vi "RT Main.vi"() -> ()   [LabVIEW 2014]
uses:
  <vilib>/NI/cRIO Wfm/cRIO Wfm.lvlib
  <vilib>/NI/cRIO Wfm/AcqRead(Wfm).vi
  <vilib>/rvi/interface/nirviOpenFPGA/nirviOpenFPGA.xnode
  <vilib>/rvi/interface/nirviMethod/nirviMethod.xnode
  <vilib>/FPGAPlugInAG/Dynamic/niLvFpga_Reset_Dynamic.vi
  <vilib>/FPGAPlugInAG/Dynamic/niLvFpga_Run_Dynamic.vi
  <vilib>/rvi/interface/nirviCloseFPGA/nirviCloseFPGA.xnode
  <vilib>/addons/Sound and Vibration/svt_Calibration/SoundVib_Calibration.lvlib
  <vilib>/addons/Sound and Vibration/svt_Calibration/SVL Scale Voltage to EU (N Ch - 1 Info).vi
  <vilib>/addons/_NISVFA/_Baseband FFT/SVFA Power Spectrum (N Ch).vi
  <vilib>/addons/_NISVFA/_Zoom FFT/SVFA Zoom Power Spectrum (N Ch).vi
  <vilib>/addons/_NISVFA/_Subset FFT/SVFA Power Spectrum Subset (N Ch).vi
  <vilib>/addons/_NISVFA/_Baseband FFT/SVFA FFT Spectrum (Mag-Phase) (N Ch).vi
  <vilib>/addons/_NISVFA/_Zoom FFT/SVFA Zoom FFT Spectrum (Mag-Phase) (N Ch).vi
  <vilib>/addons/_NISVFA/_Subset FFT/SVFA FFT Spectrum Subset (Mag-Phase) (N Ch).vi
  <vilib>/addons/_NISVFA/_Baseband FFT/SVFA Power Spectral Density (N Ch).vi
  <vilib>/addons/_NISVFA/_Zoom FFT/SVFA Zoom Power Spectral Density (N Ch).vi
  <vilib>/addons/_NISVFA/_Subset FFT/SVFA Power Spectral Density Subset (N Ch).vi
  <vilib>/NI/cRIO Wfm/ChannelConfig.ctl
  <vilib>/NI/cRIO Wfm/DynamicFPGAref.ctl
  <vilib>/FPGAPlugInAG/Dynamic/niLvFpga_Close_Dynamic.vi
  FPGA Bitfiles/SOMHands-OnExerc_FPGATarget_FPGAMainSPIAPI_7cwEv4E7lq8.lvbitx
  <vilib>/FPGAPlugInAG/sbRIO-9651/niLvFpga_Open_sbRIO-9651.vi
  <vilib>/rvi/interface/common/dynamic/niFpgaDynamicAddResources.vi
  <vilib>/addons/_NISVFA/_Shared subVIs/Controls/svc_Window.ctl
  <vilib>/addons/_NISVFA/_Shared subVIs/Controls/svc_Engineering Units Text Ring.ctl
  <vilib>/addons/_NISVFA/_Shared subVIs/Controls/svc_Weighting Filter Text Ring.ctl
  <vilib>/addons/_NISVFA/_Shared subVIs/Controls/svc_Channel Info.ctl
panel:
  in  "channel info":T1={"sensor sensitivity [mV/EU]"=1000.0, "engineering units"=1, "dB reference [EU]"=1.0, "custom label"="EU", "weighting filter"=0, "pregain [dB]"=0.0} {"pregain [dB]" format="%.2f"; "weighting filter" items=["Linear", "A-weighting", "B-weighting", "C-weighting", "ITU-R 468-4", "Dolby", "CCITT", "C-message", "Wb", "Wc", "Wd", "We", "Wf", "Wh", "Wj", "Wk", "Wm", "AES17 20 kHz lowpass", "AES17 40 kHz lowpass", "AES17 20 kHz highpass", "AES17 40 kHz highpass"]; "dB reference [EU]" format="%^.1e"; "engineering units" items=["custom..."=0, "V"=1, "A"=21, "Pa"=2, "N"=20, "g"=3, "m/s^2"=4, "m/s"=5, "m"=6, "mm/s"=12, "mm"=13, "micron/s"=14, "micron"=15, "in/s^2"=7, "in/s"=8, "in"=9, "mil/s"=10, "mil"=11, "rad/s^2"=16, "rad/s"=17, "rad"=18, "deg/s^2"=26, "deg/s"=27, "deg"=28, "RPM"=22, "cycle/s^2"=23, "Hz"=24, "cycle"=25, "strain"=19]; "sensor sensitivity [mV/EU]" format="%.2f"}
  in  "scan rate [S/s]":u32=25000
  in  "quit":bool
  in  "window":T4=1 items=["None"=0, "Hanning"=1, "Hamming"=2, "Blackman-Harris"=3, "Exact Blackman"=4, "Blackman"=5, "Flat Top"=6, "4 Term B-Harris "=7, "7 Term B-Harris"=8, "Low Sidelobe"=9, "Force"=64, "Exponential"=65, "Blackman Nuttall"=11, "Triangle"=30, "Bartlett-Hanning"=31, "Bohman"=32, "Parzen"=33, "Welch"=34, "Kaiser"=60, "Dolph-Chebyshev"=61, "Gaussian"=62]
  in  "Graph Tab Control":T5(tab)
  out "Power spectrum":cluster{"f0":dbl, "df":dbl, "magnitude":dbl[]}[](graph)
  out "Phase":cluster{"f0":dbl, "df":dbl, "phase":dbl[]}[](graph)
  out "Magnitude":cluster{"f0":dbl, "df":dbl, "magnitude":dbl[]}[](graph)
  out "PSD":cluster{"f0":dbl, "df":dbl, "magnitude":dbl[]}[](graph)
  in  "dB On":bool=TRUE
  in  "FFT Type":enum32{"Baseband", "Zoom", "Subset"}(tab)
  out "frequency resolution [Hz]":dbl=50.0 format="%.2f"
  out "time record [ms]":dbl=20.0 format="%.2f"
  in  "zoom settings":T6={"frequency range"={"start frequency"=500.0, "stop frequency"=2000.0}, "window"=enum."Hanning", "number of lines"=400, "% overlap"=0.0} {"% overlap" min=0.0 max=99.0 step=10.0 format="%.2f"; "number of lines" min=1 step=1; "frequency range"."stop frequency" min=0.0 format="%.2f"; "frequency range"."start frequency" min=0.0 format="%.2f"}
  out "zoom FFT":dbl=2.500000055879356 format="%.2f"
  out "baseband FFT":dbl=50.0 format="%.2f"
  out "frequency resolution [Hz] Subset":dbl format="%.2f"
  out "time record [ms] Subset":dbl format="%.2f"
  in  "frequency range 2":T7={"start frequency"=200.0, "stop frequency"=2000.0} {"stop frequency" min=0.0 format="%.2f"; "start frequency" min=0.0 format="%.2f"}
  in  "number of samples":i32=2000 min=128
  out "averages completed":dbl
  out "done":bool
  in  "averaging mode":T8(ring)=enum."RMS averaging"
  in  "number of averages":u32=10
  in  "linear mode":enum16{"One shot", "Auto restart"}(ring)=enum."Auto restart"
  in  "weighting mode":enum16{"Linear", "Exponential"}(ring)=enum."Exponential"
  in  "restart 2":bool
  in  "Samples per Channel":i32=1000
  # "Channel Settings"
  # "Averaging Settings"
  # "Analysis Settings"
  # "VI Controls"
  # "Increase number of samples to improve frequency resolution (for a given sampling frequency)"
  # "frequency resolution [Hz]"
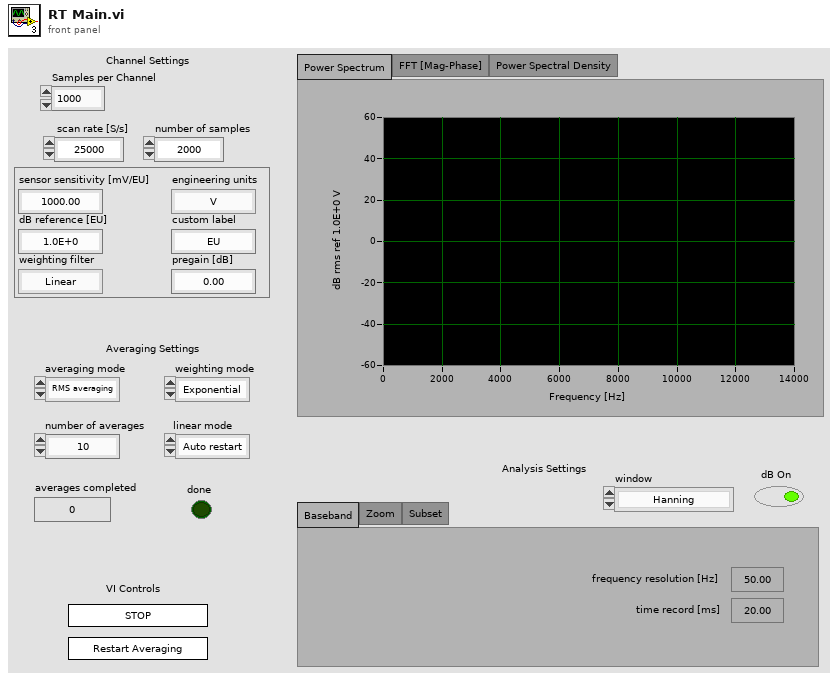
[diagram p1: front panel]
types:
  T1 = typedef "svc_Channel Info.ctl" = cluster{"sensor sensitivity [mV/EU]":dbl, "engineering units":T2, "dB reference [EU]":dbl, "custom label":string, "weighting filter":T3, "pregain [dB]":dbl}
  T2 = typedef "svc_Engineering Units Text Ring.ctl" = u16
  T3 = typedef "svc_Weighting Filter Text Ring.ctl" = u16
  T4 = typedef "svc_Window.ctl" = u32
  T5 = enum32{"Power Spectrum", "FFT [Mag-Phase]", "Power Spectral Density"}
  T6 = cluster{"frequency range":cluster{"start frequency":dbl, "stop frequency":dbl}, "window":enum16{"None ", "Hanning", "Hamming", "Blackman-Harris", "Exact Blackman", "Blackman", "Flat Top", "4 Term B-Harris ", "7 Term B-Harris", "Low Sidelobe"}, "number of lines":i32, "% overlap":dbl}
  T7 = cluster{"start frequency":dbl, "stop frequency":dbl}
  T8 = enum16{"No averaging", "Vector averaging", "RMS averaging", "Peak hold"}
  T9 = typedef "cRIO Wfm.lvlib/ChannelConfig.ctl" = cluster{"Channel Name":string, "Sensitivity mV_EU":dbl, "EU":string, "dB Ref EU":dbl}[]
  T10 = typedef "cRIO Wfm.lvlib/SamplingInfo.ctl" = cluster{"Number of Channels":i32, "Actual Samp Rate":dbl, "Chan Name Array":string[], "EU Chan Array":string[], "dB Ref Chan Array":dbl[]}
  T11 = typedef "cRIO Wfm.lvlib/DynamicFPGAref.ctl" = refnum<k20>
  T12 = cluster{"averaging mode":enum16{"No averaging", "Vector averaging", "RMS averaging", "Peak hold"}, "weighting mode":enum16{"Linear", "Exponential"}, "number of averages":u32, "linear mode":enum16{"One shot", "Auto restart"}}
  T13 = cluster{"dB On (T)":bool, "unwrap phase (F)":bool, "convert to degree (T)":bool}
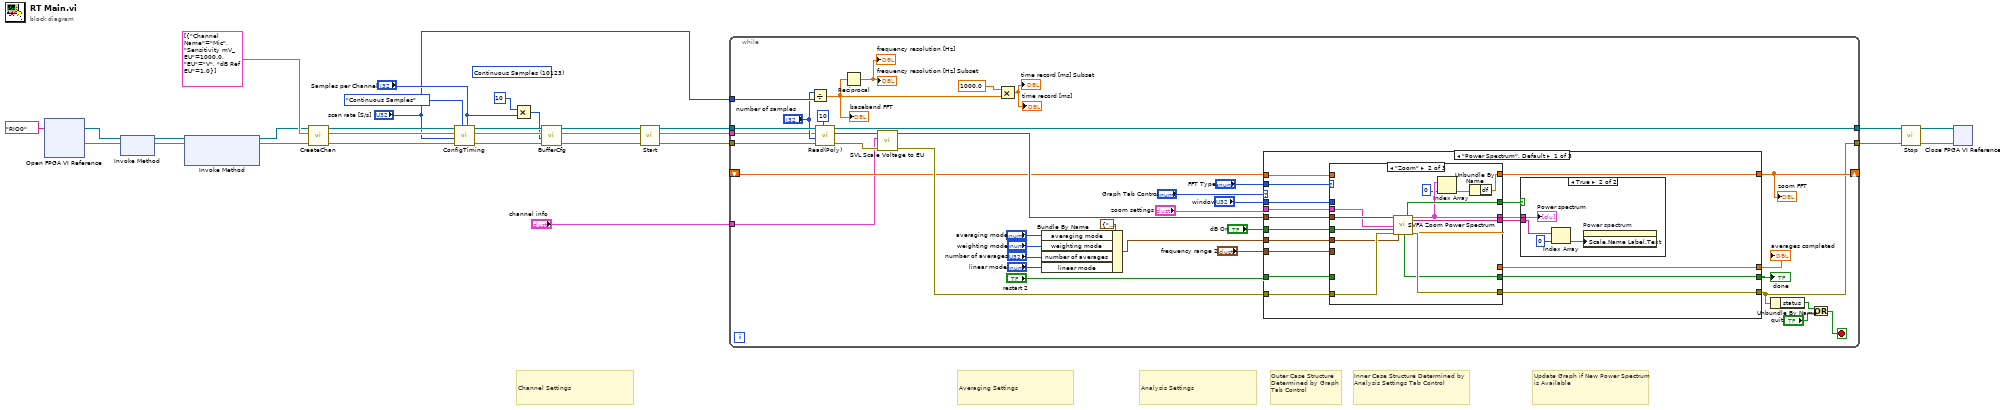
[diagram p0: block diagram]
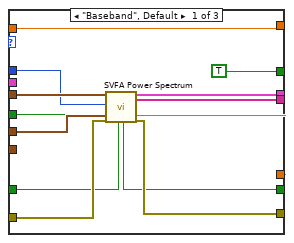
[diagram p3: hidden frame]
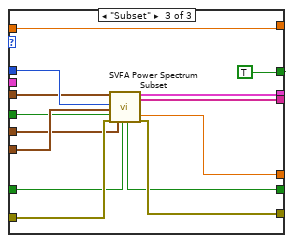
[diagram p4: hidden frame]
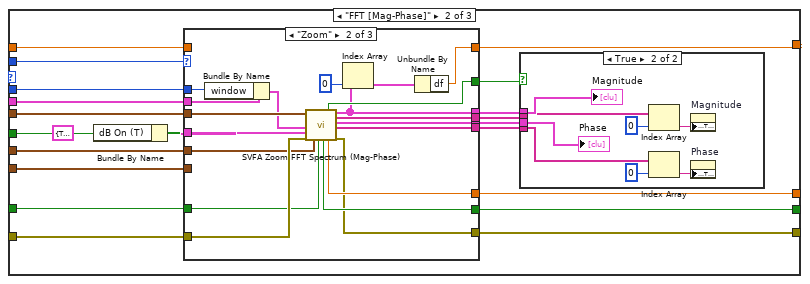
[diagram p5: hidden frame]
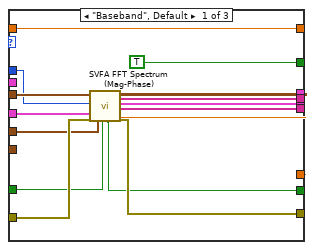
[diagram p7: hidden frame]
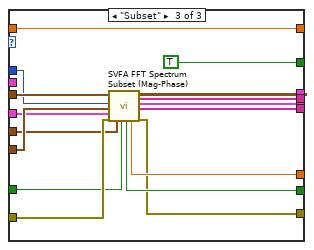
[diagram p8: hidden frame]
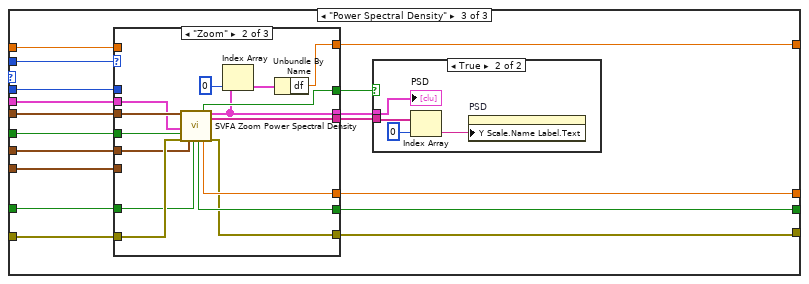
[diagram p9: hidden frame]
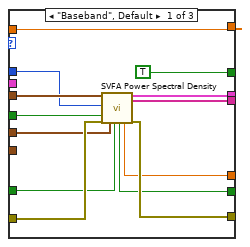
[diagram p11: hidden frame]
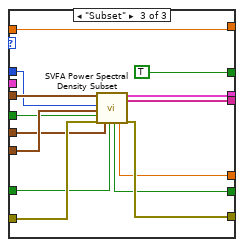
[diagram p12: hidden frame]
diagram:
  (unwired) 10123 items=["Finite Samples"=10178, "Continuous Samples"=10123] ("sample mode")
  # "Channel Settings"
  # "Update Graph if New Power Spectrum is Available"
  # "Inner Case Structure Determined by Analysis Settings Tab Control"
  # "Analysis Settings"
  # "Outer Case Structure Determined by Graph Tab Control"
  # "Averaging Settings"
  n1 = xnode "Open FPGA VI Reference"("resource name"=tag "RIO0") -> ("FPGA VI Reference Out"=w17:refnum<k20>, "error out"=w18:errorcluster)  [unwired: 1 in]
  n2 = xnode "Invoke Method"("FPGA VI Reference In"=w17, "error in"=w18) -> ("FPGA VI Reference Out"=w16:refnum<k20>, "error out"=w14:errorcluster)
  n3 = xnode "Invoke Method"("FPGA VI Reference In"=w16, "error in"=w14) -> ("FPGA VI Reference Out"=w2:refnum<k20>, "error out"=w15:errorcluster)  [unwired: 1 in]
  n4 = call <vilib>:"CreateChan.vi"("error in"=w15, "Channel Info"=T9 [{"Channel Name"="Mic", "Sensitivity mV_EU"=1000.0, "EU"="V", "dB Ref EU"=1.0}], "Dynamic FPGA Ref"=w2) -> ("error out"=w1:errorcluster, "Sampling Info"=w24:T10, "Dynamic FPGA Ref Out"=w30:T11)  [unwired: 6 in]
  n5 = call <vilib>:"ConfigTiming.vi"("Samples per Channel"="Samples per Channel", "Sample Mode"=enum16{"Finite Samples", "Continuous Samples"}."Continuous Samples", "error in"=w1, "Sample Rate"="scan rate [S/s]", "Sampling Info In"=w24, "Dynamic FPGA Ref"=w30) -> ("error out"=w20:errorcluster, "Sampling Info Out"=w25:T10, "Dynamic FPGA Ref Out"=w29:T11)  [unwired: 2 in, 1 out]
  n6 = Multiply(x=10, y="Samples per Channel") -> (x*y=w21:i32)
  n7 = call <vilib>:"BufferCfg.vi"("error in"=w20, "Buffer Size [Samps per Chan]"=w21, "Sampling Info In"=w25, "Dynamic FPGA Ref"=w29) -> ("error out"=w19:errorcluster, "Sampling Info Out"=w23:T10, "Dynamic FPGA Ref Out"=w28:T11)  [unwired: 4 in, 1 out]
  n8 = call <vilib>:"Start.vi"("error in"=w19, "Sampling Info In"=w23, "Dynamic FPGA Ref"=w28) -> ("error out"=w5:errorcluster, "Sampling Info Out"=w4:T10, "Dynamic FPGA Ref Out"=w6:T11)  [unwired: 6 in]
  n9 = while {
    tunnel: [w33] -> w8
    shift-right: [w54] -> _
    shift-left: _ -> [w57]
    tunnel: [w49] -> w9
    tunnel: w6 -> [w48]
    tunnel: "scan rate [S/s]" -> [w47]
    tunnel: w5 -> [w44]
    tunnel: "channel info" -> [w35]
    tunnel: w4 -> [w31]
    stop <- w66 stop-if-true
    n10 = Divide(x="number of samples", y=w47) -> (x/y=w55:dbl)
    "baseband FFT" <- w55
    n11 = call-poly <vilib>:"Read(Poly).vi"("Poll Time (ms)"=u32 10, "error in"=w44, "Samps Read per Chan"="number of samples", "Sampling Info"=w31, "Dynamic FPGA Ref"=w48) -> ("error out"=w45:errorcluster, "Wfm Data"=w50:waveform(sgl)[], "Dynamic FPGA Ref Out"=w49:T11)  [unwired: 3 in, 1 out]
    n12 = Reciprocal(x=w55) -> (1/x=→"frequency resolution [Hz]" →"frequency resolution [Hz] Subset":dbl)
    n13 = call-poly <vilib>:"SVL Scale Voltage to EU.vi"("error in (no error)"=w45, "channel info"=w35, "signals [V]"=w50) -> ("error out"=w65:errorcluster, "scaled signals [EU]"=w64:waveform(dbl)[])  [unwired: 6 in, 1 out]
    n14 = Multiply(x=1000.0 ("y"), y=w55) -> (x*y=→"time record [ms]" →"time record [ms] Subset":dbl)
    n15 = Bundle By Name(cluster=T12 {"averaging mode"=enum."RMS averaging", "weighting mode"=enum."Exponential", "number of averages"=10, "linear mode"=enum."Auto restart"} ("averaging parameters"), "averaging mode"="averaging mode", "weighting mode"="weighting mode", "number of averages"="number of averages", "linear mode"="linear mode") -> (w38:T12)
    n16 = case shown="\"Power Spectrum\", Default" "Graph Tab Control" {
      tunnel: w65 -> [w83 w150 w224]
      tunnel: w64 -> [w84 w149 w225]
      tunnel: [w82 w148 w223] -> w33
      tunnel: "window" -> [w81 w132 w222]
      tunnel: w38 -> [w80 w147 w221]
      tunnel: "restart 2" -> [w79 w146 w209]
      tunnel: [w77 w145 w220] -> w36
      tunnel: [w76 w144 w219] -> w37
      tunnel: "dB On" -> [w75 w142 w213]
      tunnel: "FFT Type" -> [w73 w137 w215]
      tunnel: [w72 w134 w212] -> w54
      tunnel: w57 -> [w70 w133 w211]
      tunnel: "zoom settings" -> [w69 w136 w214]
      tunnel: "frequency range 2" -> [w68 w131 w210]
      frame "Power Spectrum", Default {
        n17 = case shown="\"Zoom\"" w73 {
          tunnel: w84 -> [w101 w115 w127]
          tunnel: w83 -> [w100 w114 w126]
          tunnel: [w99 w113 w124] -> w82
          tunnel: w81 -> [w98 _ w128]
          tunnel: w80 -> [w97 w102 w116]
          tunnel: w79 -> [w96 _ w118]
          tunnel: [w95 w104 w125] -> w78
          tunnel: [w94 w108 w119] -> w77
          tunnel: [w93 w107 w120] -> w76
          tunnel: w75 -> [w92 w106 w117]
          tunnel: [w91 w110 w123] -> w74
          tunnel: [w89 w112 w121] -> w72
          tunnel: [TRUE ("new spectrum available") w111 TRUE ("new spectrum available")] -> w71
          tunnel: w70 -> [w89 _ w121]
          tunnel: w69 -> [_ w109 _]
          tunnel: w68 -> [_ _ w129]
          frame "Baseband", Default {
            n18 = call-poly <vilib>:"SVFA Power Spectrum.vi"("scaled signals [EU]"=w101, "window"=w98, "dB On (T)"=w92, "error in (no error)"=w100, "averaging parameters"=w97, "restart averaging (F)"=w96) -> ("averaging done"=w94:bool, "averages completed"=w93:dbl, "power spectra [dB EU]"=w95:cluster{"f0":dbl, "df":dbl, "magnitude":dbl[]}[], "unit labels"=w91:string[], "error out"=w99:errorcluster)  [unwired: 8 in, 1 out]
          }
          frame "Zoom" {
            n19 = call-poly <vilib>:"SVFA Zoom Power Spectrum.vi"("scaled signals [EU]"=w115, "zoom settings"=w109, "dB On (T)"=w106, "error in (no error)"=w114, "averaging parameters"=w102) -> ("averaging done"=w108:bool, "new spectrum available"=w111:bool, "averages completed"=w107:dbl, "power spectra [dB EU]"=w104:cluster{"f0":dbl, "df":dbl, "magnitude":dbl[]}[], "unit labels"=w110:string[], "error out"=w113:errorcluster)  [unwired: 8 in, 1 out]
            n20 = Index Array(array=w104, index=0) -> (element=w105:cluster{"f0":dbl, "df":dbl, "magnitude":dbl[]})
            n21 = Unbundle By Name(w105) -> ("df"=w112:dbl)
          }
          frame "Subset" {
            n22 = call-poly <vilib>:"SVFA Power Spectrum Subset.vi"("scaled signals [EU]"=w127, "window"=w128, "frequency range"=w129, "dB On (T)"=w117, "error in (no error)"=w126, "averaging parameters"=w116, "restart averaging (F)"=w118) -> ("averaging done"=w119:bool, "averages completed"=w120:dbl, "power spectra [dB EU]"=w125:cluster{"f0":dbl, "df":dbl, "magnitude":dbl[]}[], "unit labels"=w123:string[], "error out"=w124:errorcluster)  [unwired: 7 in, 1 out]
          }
        }
        n23 = case shown="True" w71 {
          tunnel: w78 -> [_ w88]
          tunnel: w74 -> [_ w87]
          frame False {
          }
          frame True {
            n24 = Index Array(array=w87, index=0) -> (element=w85:string)
            n25 = property on="Power spectrum" class="WFGraph (strict)"("Y Scale.Name Label.Text"=w85) -> ()  [unwired: 2 in, 2 out]
            "Power spectrum" <- w88
          }
        }
      }
      frame "FFT [Mag-Phase]" {
        n26 = Bundle By Name(cluster=T13 {"dB On (T)"=TRUE, "unwrap phase (F)"=FALSE, "convert to degree (T)"=TRUE} ("view"), "dB On (T)"=w142) -> (w141:T13)
        n27 = case shown="\"Zoom\"" w137 {
          tunnel: w150 -> [w173 w189 w207]
          tunnel: w149 -> [w172 w192 w208]
          tunnel: [w171 w185 w202] -> w148
          tunnel: w147 -> [w170 w188 w194]
          tunnel: w146 -> [w169 w179 w205]
          tunnel: [w168 w187 w204] -> w145
          tunnel: [w167 w186 w203] -> w144
          tunnel: w132 -> [w166 w177 w193]
          tunnel: [w165 w176 w201] -> w143
          tunnel: w141 -> [w164 w190 w197]
          tunnel: [w163 w183 w195] -> w130
          tunnel: [w162 w184 w198] -> w140
          tunnel: [w161 w182 w200] -> w138
          tunnel: w136 -> [_ w191 _]
          tunnel: [TRUE ("new spectrum available") w181 TRUE ("new spectrum available")] -> w135
          tunnel: [w159 w180 w196] -> w134
          tunnel: w133 -> [w159 _ w196]
          tunnel: w131 -> [_ _ w206]
          frame "Baseband", Default {
            n28 = call-poly <vilib>:"SVFA FFT Spectrum (Mag-Phase).vi"("scaled signals [EU]"=w172, "window"=w166, "view"=w164, "error in (no error)"=w173, "averaging parameters"=w170, "restart averaging (F)"=w169) -> ("averaging done"=w168:bool, "averages completed"=w167:dbl, "magnitudes [dB EU]"=w165:cluster{"f0":dbl, "df":dbl, "magnitude":dbl[]}[], "magnitude unit labels"=w162:string[], "phases [degrees]"=w163:cluster{"f0":dbl, "df":dbl, "phase":dbl[]}[], "phase unit labels"=w161:string[], "error out"=w171:errorcluster)  [unwired: 6 in, 1 out]
          }
          frame "Zoom" {
            n29 = Bundle By Name(cluster=w191, "window"=w177) -> (w178:T6)
            n30 = call-poly <vilib>:"SVFA Zoom FFT Spectrum (Mag-Phase).vi"("scaled signals [EU]"=w192, "zoom settings"=w178, "view"=w190, "error in (no error)"=w189, "averaging parameters"=w188, "restart averaging (F)"=w179) -> ("averaging done"=w187:bool, "new spectrum available"=w181:bool, "averages completed"=w186:dbl, "magnitudes [dB EU]"=w176:cluster{"f0":dbl, "df":dbl, "magnitude":dbl[]}[], "magnitude unit labels"=w184:string[], "phases [degrees]"=w183:cluster{"f0":dbl, "df":dbl, "phase":dbl[]}[], "phase unit labels"=w182:string[], "error out"=w185:errorcluster)  [unwired: 5 in, 1 out]
            n31 = Index Array(array=w176, index=0) -> (element=w175:cluster{"f0":dbl, "df":dbl, "magnitude":dbl[]})
            n32 = Unbundle By Name(w175) -> ("df"=w180:dbl)
          }
          frame "Subset" {
            n33 = call-poly <vilib>:"SVFA FFT Spectrum Subset (Mag-Phase).vi"("scaled signals [EU]"=w208, "window"=w193, "frequency range"=w206, "view"=w197, "error in (no error)"=w207, "averaging parameters"=w194, "restart averaging (F)"=w205) -> ("averaging done"=w204:bool, "averages completed"=w203:dbl, "magnitudes [dB EU]"=w201:cluster{"f0":dbl, "df":dbl, "magnitude":dbl[]}[], "magnitude unit labels"=w198:string[], "phases [degrees]"=w195:cluster{"f0":dbl, "df":dbl, "phase":dbl[]}[], "phase unit labels"=w200:string[], "error out"=w202:errorcluster)  [unwired: 5 in, 1 out]
          }
        }
        n34 = case shown="True" w135 {
          tunnel: w143 -> [_ w158]
          tunnel: w140 -> [_ w153]
          tunnel: w138 -> [_ w156]
          tunnel: w130 -> [_ w157]
          frame False {
          }
          frame True {
            n35 = Index Array(array=w153, index=0) -> (element=w151:string)
            n36 = Index Array(array=w156, index=0) -> (element=w154:string)
            n37 = property on="Magnitude" class="WFGraph (strict)"("Y Scale.Name Label.Text"=w151) -> ()  [unwired: 2 in, 2 out]
            n38 = property on="Phase" class="WFGraph (strict)"("Y Scale.Name Label.Text"=w154) -> ()  [unwired: 2 in, 2 out]
            "Magnitude" <- w158
            "Phase" <- w157
          }
        }
      }
      frame "Power Spectral Density" {
        n39 = case shown="\"Zoom\"" w215 {
          tunnel: w225 -> [w242 w257 w270]
          tunnel: w224 -> [w241 w256 w263]
          tunnel: [w240 w249 w271] -> w223
          tunnel: w222 -> [w239 _ w262]
          tunnel: w221 -> [w238 w253 w259]
          tunnel: w209 -> [w237 w252 w258]
          tunnel: [w236 w251 w264] -> w220
          tunnel: [w235 w250 w265] -> w219
          tunnel: [w234 w245 w268] -> w218
          tunnel: [w233 w248 w267] -> w217
          tunnel: [TRUE ("new spectrum available") w247 TRUE ("new spectrum available")] -> w216
          tunnel: w214 -> [_ w255 _]
          tunnel: w213 -> [w230 w254 w260]
          tunnel: [w232 w246 w269] -> w212
          tunnel: w211 -> [w232 _ w269]
          tunnel: w210 -> [_ _ w261]
          frame "Baseband", Default {
            n40 = call-poly <vilib>:"SVFA Power Spectral Density.vi"("scaled signals [EU]"=w242, "window"=w239, "dB On (F)"=w230, "error in (no error)"=w241, "averaging parameters"=w238, "restart averaging (F)"=w237) -> ("averaging done"=w236:bool, "averages completed"=w235:dbl, "power spectral densities [EU^2 rms / Hz]"=w234:cluster{"f0":dbl, "df":dbl, "magnitude":dbl[]}[], "unit labels"=w233:string[], "error out"=w240:errorcluster)  [unwired: 8 in, 1 out]
          }
          frame "Zoom" {
            n41 = call-poly <vilib>:"SVFA Zoom Power Spectral Density.vi"("scaled signals [EU]"=w257, "zoom settings"=w255, "dB On (T)"=w254, "error in (no error)"=w256, "averaging parameters"=w253, "restart averaging (F)"=w252) -> ("averaging done"=w251:bool, "new spectrum available"=w247:bool, "averages completed"=w250:dbl, "power spectral densities [EU^2 rms / Hz]"=w245:cluster{"f0":dbl, "df":dbl, "magnitude":dbl[]}[], "unit labels"=w248:string[], "error out"=w249:errorcluster)  [unwired: 7 in, 1 out]
            n42 = Index Array(array=w245, index=0) -> (element=w244:cluster{"f0":dbl, "df":dbl, "magnitude":dbl[]})
            n43 = Unbundle By Name(w244) -> ("df"=w246:dbl)
          }
          frame "Subset" {
            n44 = call-poly <vilib>:"SVFA Power Spectral Density Subset.vi"("scaled signals [EU]"=w270, "window"=w262, "frequency range"=w261, "dB On (T)"=w260, "error in (no error)"=w263, "averaging parameters"=w259, "restart averaging (F)"=w258) -> ("averaging done"=w264:bool, "averages completed"=w265:dbl, "power spectral densities [EU^2 rms / Hz]"=w268:cluster{"f0":dbl, "df":dbl, "magnitude":dbl[]}[], "unit labels"=w267:string[], "error out"=w271:errorcluster)  [unwired: 7 in, 1 out]
          }
        }
        n45 = case shown="True" w216 {
          tunnel: w218 -> [_ w229]
          tunnel: w217 -> [_ w228]
          frame False {
          }
          frame True {
            n46 = Index Array(array=w228, index=0) -> (element=w226:string)
            n47 = property on="PSD" class="WFGraph (strict)"("Y Scale.Name Label.Text"=w226) -> ()  [unwired: 2 in, 2 out]
            "PSD" <- w229
          }
        }
      }
    }
    "zoom FFT" <- w54
    "averages completed" <- w37
    "done" <- w36
    n48 = Unbundle By Name(w33) -> ("status"=w63:bool)
    n49 = Or(x=w63, y="quit") -> (x .or. y?=w66:bool)
  }
  n50 = call <vilib>:"Stop.vi"("error in"=w8, "Dynamic FPGA Ref"=w9) -> ("error out"=w12:errorcluster, "Dynamic FPGA Ref Out"=w13:T11)  [unwired: 8 in]
  n51 = xnode "Close FPGA VI Reference"("FPGA VI Reference In"=w13, "error in"=w12) -> ()  [unwired: 1 out]
